vi "Elevator Encoder Config.vi"(0 "Number Samples to Average":u8=1, 1 "Minimum Rate":dbl=20.0, 2 "DistancePerCount":dbl=1.0, 3 "Decoding Type":T2=enum."4x", 9 "Channel B":T1, 11 "Channel A":T1) -> ()   [LabVIEW 2012]
uses:
  <vilib>/Rock Robotics/WPI/Encoder/WPI_EncoderType.ctl
  <vilib>/Rock Robotics/SystemInterfaces/DIO/FPGA_DIOChannel.ctl
  <vilib>/Rock Robotics/WPI/Counter/WPI_CounterDigitalInputToDigitalSource.vi
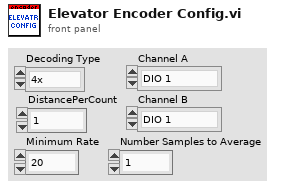
[diagram p1: front panel]
types:
  T1 = typedef "FPGA_DIOChannel.ctl" = enum8{"DIO 1", "DIO 2", "DIO 3", "DIO 4", "DIO 5", "DIO 6", "DIO 7", "DIO 8", "DIO 9", "DIO 10", "DIO 11", "DIO 12", "DIO 13", "DIO 14", "Invalid"}
  T2 = typedef "WPI_EncoderType.ctl" = enum16{"1x", "2x", "4x"}
  T3 = typedef "WPI_DigitalInputDevRef.ctl" = cluster{"DevStatus":errorcluster, "DIO Channel":T1, "Digital Module":T4}
  T4 = typedef "FPGA_TypedefDigitalModule.ctl" = enum16{"Digital Module 1", "Digital Module 2"}
  T5 = typedef "FPGA_CounterEncoderSourceConvertionLVSourceType.ctl" = cluster{"DevStatus":errorcluster, "AnalogTriggerMode?":bool, "DigitalMode":cluster{"Digital Module":T4, "DIO Channel":T6}, "AnalogTriggerMode":cluster{"AnalogTriggerIndex":T7, "OutputType":T8}}
  T6 = typedef "FPGA_DIODigitalSourceChannel.ctl" = enum8{"DIO 1", "DIO 2", "DIO 3", "DIO 4", "DIO 5", "DIO 6", "DIO 7", "DIO 8", "DIO 9", "DIO 10", "DIO 11", "DIO 12", "DIO 13", "DIO 14", "Disabled"}
  T7 = typedef "FPGA_AnalogTriggerIndex.ctl" = enum8{"Trig 0", "Trig 1", "Trig 2", "Trig 3", "Trig 4", "Trig 5", "Trig 6", "Trig 7", "Invalid"}
  T8 = typedef "FPGA_AnalogTriggerOutType.ctl" = enum16{"InWindow", "TriggerState", "Rising", "Falling"}
  T9 = typedef "WPI_EncoderDevRef.ctl" = cluster{"DevStatus":errorcluster, "EncoderIndex":T10, "CounterIndex":T11, "DistancePerCount":dbl, "Decoding Type":T2}
  T10 = typedef "FPGA_EncoderIdx.ctl" = enum8{"Enc 0", "Enc 1", "Enc 2", "Enc 3", "Invalid"}
  T11 = typedef "FPGA_CounterCtrSystemIndex.ctl" = enum8{"Ctr 0", "Ctr 1", "Ctr 2", "Ctr 3", "Ctr 4", "Ctr 5", "Ctr 6", "Ctr 7", "Invalid"}
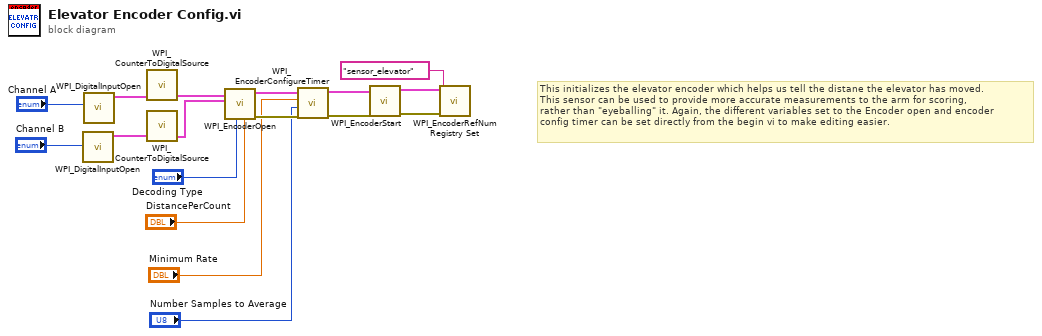
[diagram p0: block diagram]
diagram:
  # "This initializes the elevator encoder which helps us tell the distane the elevator has moved. \nThis sensor can be used to provide more accurate measurements to the arm for scoring, \nrather than \"eyeballing\" it. Again, the different variables set to the Encoder open and encoder \nconfig timer can be set directly from the begin vi to make editing easier."
  n1 = call <vilib>:"WPI_DigitalInputOpen.vi"("DIO Channel"="Channel B") -> ("DigitalInputDevRef"=w16:T3)  [unwired: 9 in, 1 out]
  n2 = call <vilib>:"WPI_DigitalInputOpen.vi"("DIO Channel"="Channel A") -> ("DigitalInputDevRef"=w17:T3)  [unwired: 9 in, 1 out]
  n3 = call-poly <vilib>:"WPI_CounterToDigitalSource.vi"("DigitalInputDevRef"=w17) -> ("Digital Source"=w15:T5)  [unwired: 6 in]
  n4 = call-poly <vilib>:"WPI_CounterToDigitalSource.vi"("DigitalInputDevRef"=w16) -> ("Digital Source"=w8:T5)  [unwired: 6 in]
  n5 = call <vilib>:"WPI_EncoderOpen.vi"("DistancePerCount"="DistancePerCount", "Decoding Type"="Decoding Type", "BSource"=w8, "ASource"=w15) -> ("error out"=w13:errorcluster, "EncoderDevRef"=w14:T9)  [unwired: 6 in]
  n6 = call <vilib>:"WPI_EncoderConfigureTimer.vi"("error in (no error)"=w13, "Number Samples to Average"="Number Samples to Average", "Minimum Rate"="Minimum Rate", "EncoderDevRef"=w14) -> ("error out"=w11:errorcluster, "EncoderDevRef"=w12:T9)  [unwired: 6 in]
  n7 = call <vilib>:"WPI_EncoderStart.vi"("error in (no error)"=w11, "EncoderDevRef"=w12) -> ("error out"=w9:errorcluster, "EncoderDevRef"=w10:T9)  [unwired: 8 in]
  n8 = call <vilib>:"WPI_EncoderRefNum Registry Set.vi"("error in (no error)"=w9, "refnum name"="sensor_elevator", "EncoderDevRef"=w10) -> ()  [unwired: 7 in, 2 out]
